vi "TestSwitchingBool_UserPressCaught.vi"(8 "error in (no error)":errorcluster, 11 "TestCase in":refnum<class "UITestAutoRegistration.lvclass">) -> (0 "error out":errorcluster, 3 "TestCase out":refnum<class "UITestAutoRegistration.lvclass">)   [LabVIEW 2017, in "UITestAutoRegistration.lvclass"]
uses:
  UITestAutoRegistration.lvclass
  C:/Program Files (x86)/National Instruments/LabVIEW 2017/vi.lib/addons/_JKI Toolkits/VI Tester/TestCase.llb/TestCase.lvclass
  <vilib>/addons/_JKI Toolkits/VI Tester/TestCase.llb/TestCase.lvclass
  Source/Framework/ActorEvents/AutoRegistration/AutoRegistration.lvclass
panel:
  in  "OK Button":bool
  # "Press and release switching button"
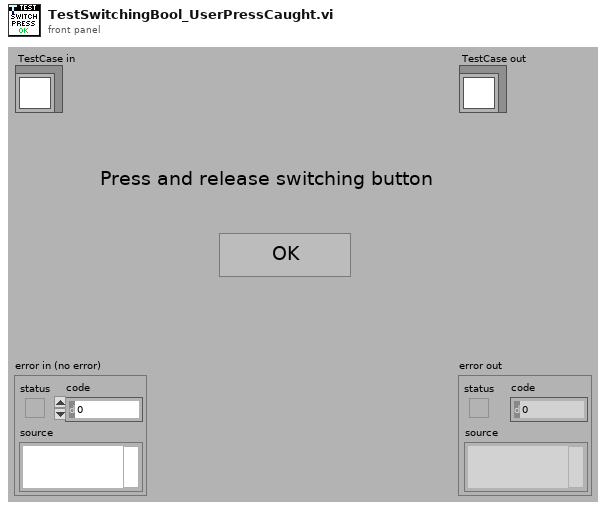
[diagram p1: front panel]
types:
  T1 = typedef "AutoRegistration.lvlib/AutoRegistration.lvclass/Auto-Event Registration Refnum.ctl" = refnum<event-registration>
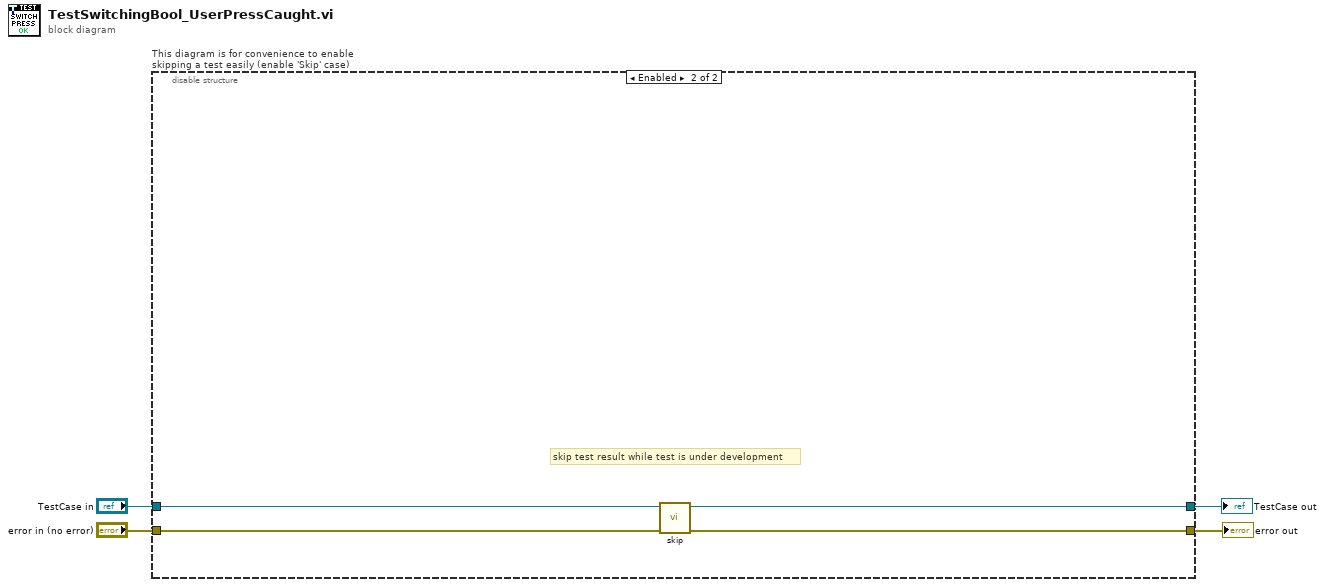
[diagram p0: block diagram]
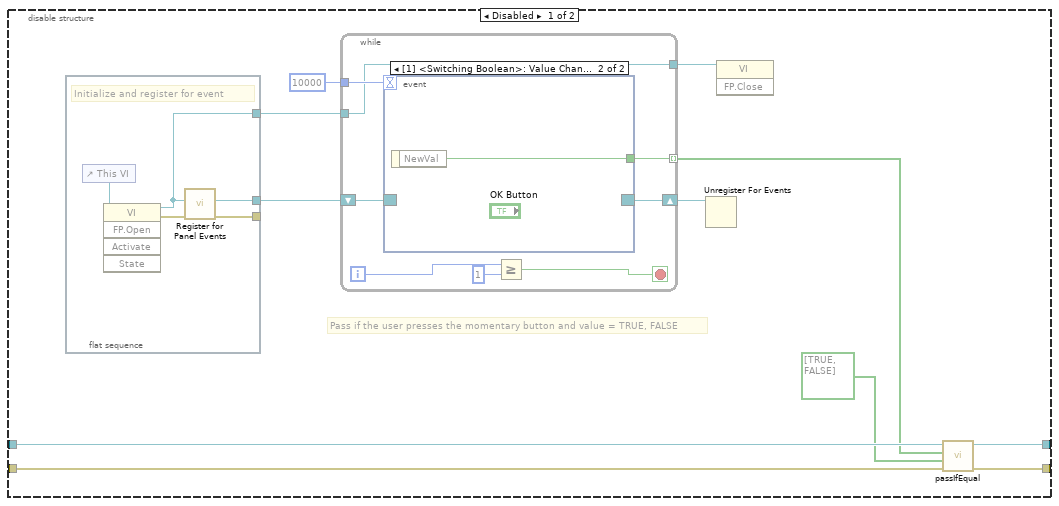
[diagram p2: hidden frame]
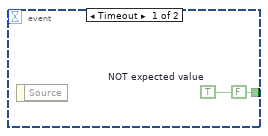
[diagram p3: hidden frame]
diagram:
  n1 = disable-structure "This diagram is for convenience to enable skipping a test easily (enable 'Skip' case)" shown="Enabled" {
    disable-tunnel: "TestCase in" -> [w15 w34]
    disable-tunnel: [w14 w32] -> w1
    disable-tunnel: [w13 w33] -> w3
    disable-tunnel: "error in (no error)" -> [w12 w31]
    frame Disabled {
      # "Pass if the user presses the momentary button and value = TRUE, FALSE"
      n2 = flat-sequence {
        tunnel: [w30] -> _
        tunnel: [w29] -> w11
        tunnel: [w26] -> w6
        frame #0 {
          # "Initialize and register for event"
          n3 = control-ref of="This VI"() -> (w28:refnum<vi>)
          n4 = invoke class="VI" method="FP.Open"(reference=w28) -> (reference out=w26:refnum<vi>, error out=w27:errorcluster)  [unwired: 4 in, 3 out]
          n5 = call "Register for Panel Events.vi"("error in (no error)"=w27, "VI Refnum (Calling VI)"=w26) -> ("error out"=w30:errorcluster, "Auto-Event Registration Refnum"=w29:T1)  [unwired: 6 in, 2 out]
        }
      }
      n6 = while {
        tunnel: 10000 -> [w21]
        tunnel: [w20] -> w8 mode=indexing
        shift-right: [w22] -> w10
        shift-left: w11 -> [w23]
        tunnel: w6 -> [w16]
        tunnel: [w16] -> w5
        i -> [w19]
        stop <- w17 stop-if-true
        n7 = event shown="[1] <Switching Boolean>: Value Change" {
          selector: w23 -> [_ _]
          dyn-events: [_ _] -> w22
          timeout: w21 -> [_ _]
          tunnel: [w24 w25] -> w20
          event Timeout {
            w24 = TRUE  # NOT expected value
            (unwired) FALSE ("NewVal")
            n8 = event-data() -> ()  [unwired: 1 in, 1 out]
          }
          event Value Change {
            n9 = event-data() -> ("NewVal"=w25:bool)  [unwired: 1 in]
          }
        }
        n10 = Greater Or Equal?(x=w19, y=1 ("x")) -> (x >= y?=w17:bool)
      }
      n11 = Unregister For Events(event registration refnum=w10) -> ()  [unwired: 1 in, 1 out]
      n12 = invoke class="VI" method="FP.Close"(reference=w5) -> ()  [unwired: 2 in, 3 out]
      n13 = call-dynamic "passIfEqual.vi"("error in (no error)"=w12, "y"=bool[] [TRUE, FALSE], "x"=w8, "TestCase in"=w15) -> ("error out"=w13:errorcluster, "TestCase out"=w14:refnum<class "UITestAutoRegistration.lvclass">)  [unwired: 6 in]
    }
    frame Enabled {
      # "skip test result while test is under development"
      n14 = call <vilib>:"skip.vi"("error in (no error)"=w31, "TestCase in"=w34) -> ("error out"=w33:errorcluster, "TestCase out"=w32:refnum<class "UITestAutoRegistration.lvclass">)  [unwired: 8 in]
    }
  }
  "error out" <- w3
  "TestCase out" <- w1
